vi "Limited Integrator (DBL).vi"(4 "initialize":bool, 5 "lower bound":dbl format="%.2f", 6 "upper bound":dbl format="%.2f", 7 "dt":dbl=1e-09 min=1e-09 format="%.6f", 9 "initial condition":dbl format="%.2f", 10 "input point":dbl format="%.2f") -> (3 "output point":dbl format="%.2f")   [LabVIEW 2020, in "NI_AdvCtrl_continuous linear.lvlib"]
doc: "LabVIEW no longer supports this VI. You can obtain similar functionality by installing the LabVIEW Simulation Module.\n\nIntegrates a continuous input signal where limits are given. The integration process is based on Euler method. dt must be positive. The result of the integration process is in between of lower bound and upper bound."
uses:
  <vilib>/addons/control/advanced/NI_AdvCtrl_continuous linear.lvlib
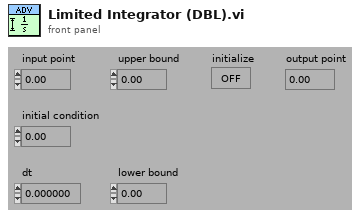
[diagram p1: front panel]
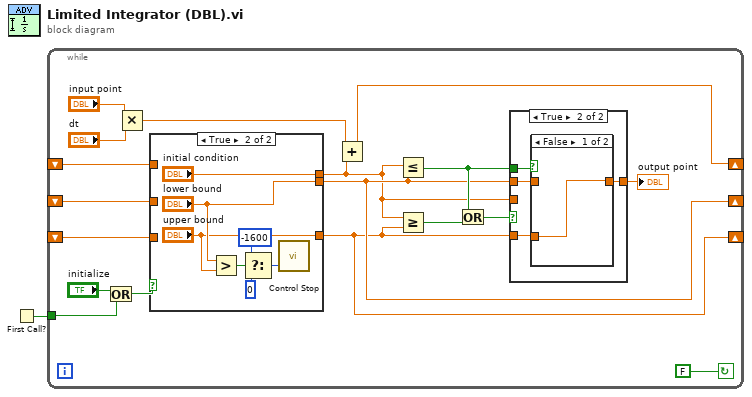
[diagram p0: block diagram]
diagram:
  n1 = First Call?() -> (First Call?: T/F=w1:bool)
  n2 = while {
    shift-left: _ -> [w5]
    shift-right: [w7] -> _
    shift-left: _ -> [w4]
    shift-right: [w6] -> _
    shift-left: _ -> [w9]
    shift-right: [w2] -> _
    tunnel: w1 -> [w18]
    stop <- FALSE continue-if-true
    n3 = Or(x="initialize", y=w18) -> (x .or. y?=w8:bool)
    n4 = Multiply(x="input point", y="dt") -> (x*y=w15:dbl)
    n5 = case shown="True" w8 {
      tunnel: [w22 "initial condition"] -> w3
      tunnel: w9 -> [w22 _]
      tunnel: [w21 "lower bound"] -> w7
      tunnel: [w20 "upper bound"] -> w6
      tunnel: w5 -> [w21 _]
      tunnel: w4 -> [w20 _]
      frame False {
      }
      frame True {
        n6 = Greater?(x="lower bound", y="upper bound") -> (0:w26:bool)
        n7 = Select(t=-1600, s=w26, f=0) -> (s? t:f=w24:i32)
        n8 = call <vilib>:"Control Stop.vi"("error"=w24) -> ()  [unwired: 2 out]
      }
    }
    n9 = Add(x=w15, y=w3) -> (x+y=w2:dbl)
    n10 = Less Or Equal?(x=w3, y=w7) -> (x <= y?=w13:bool)
    n11 = Greater Or Equal?(x=w3, y=w6) -> (x >= y?=w12:bool)
    n12 = Or(x=w13, y=w12) -> (x .or. y?=w14:bool)
    n13 = case shown="True" w14 {
      tunnel: [w30 w32] -> w11
      tunnel: w3 -> [w30 _]
      tunnel: w13 -> [_ w34]
      tunnel: w7 -> [_ w33]
      tunnel: w6 -> [_ w31]
      frame False {
      }
      frame True {
        n14 = case shown="False" w34 {
          tunnel: w33 -> [_ w36]
          tunnel: [w35 w36] -> w32
          tunnel: w31 -> [w35 _]
          frame False {
          }
          frame True {
          }
        }
      }
    }
    "output point" <- w11
  }
